vi "Enable-Disable SCISCAN Controls.vi"(7 "Enable-Disable SCISCAN Controls_Command":T2, 8 "Error In":errorcluster) -> (0 "Error Out":errorcluster)   [LabVIEW 2012]
doc: "SciScan 1.2 160622"
uses:
  Enable-Disable SCISCAN controls_Command.ctl
panel:
  out "Array":T1(array[cluster])
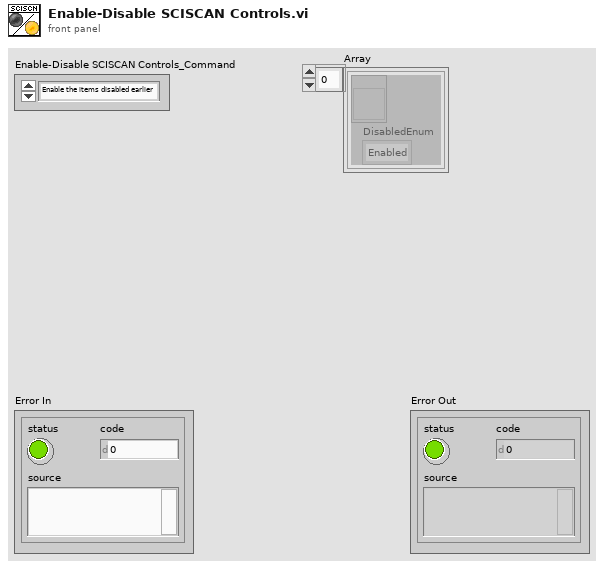
[diagram p1: front panel]
types:
  T1 = cluster{refnum<vi>, "DisabledEnum":enum8{"Enabled", "Disabled", "Disabled and Grayed Out"}}[]
  T2 = typedef "Enable-Disable SCISCAN controls_Command.ctl" = enum16{"Enable the items disabled earlier", "Disable", "Disable and Gray", "Enable all (except those in skip list)"}
  T3 = enum8{"Enabled", "Disabled", "Disabled and Grayed Out"}
  T4 = cluster{refnum<vi>, "DisabledEnum":enum8{"Enabled", "Disabled", "Disabled and Grayed Out"}}
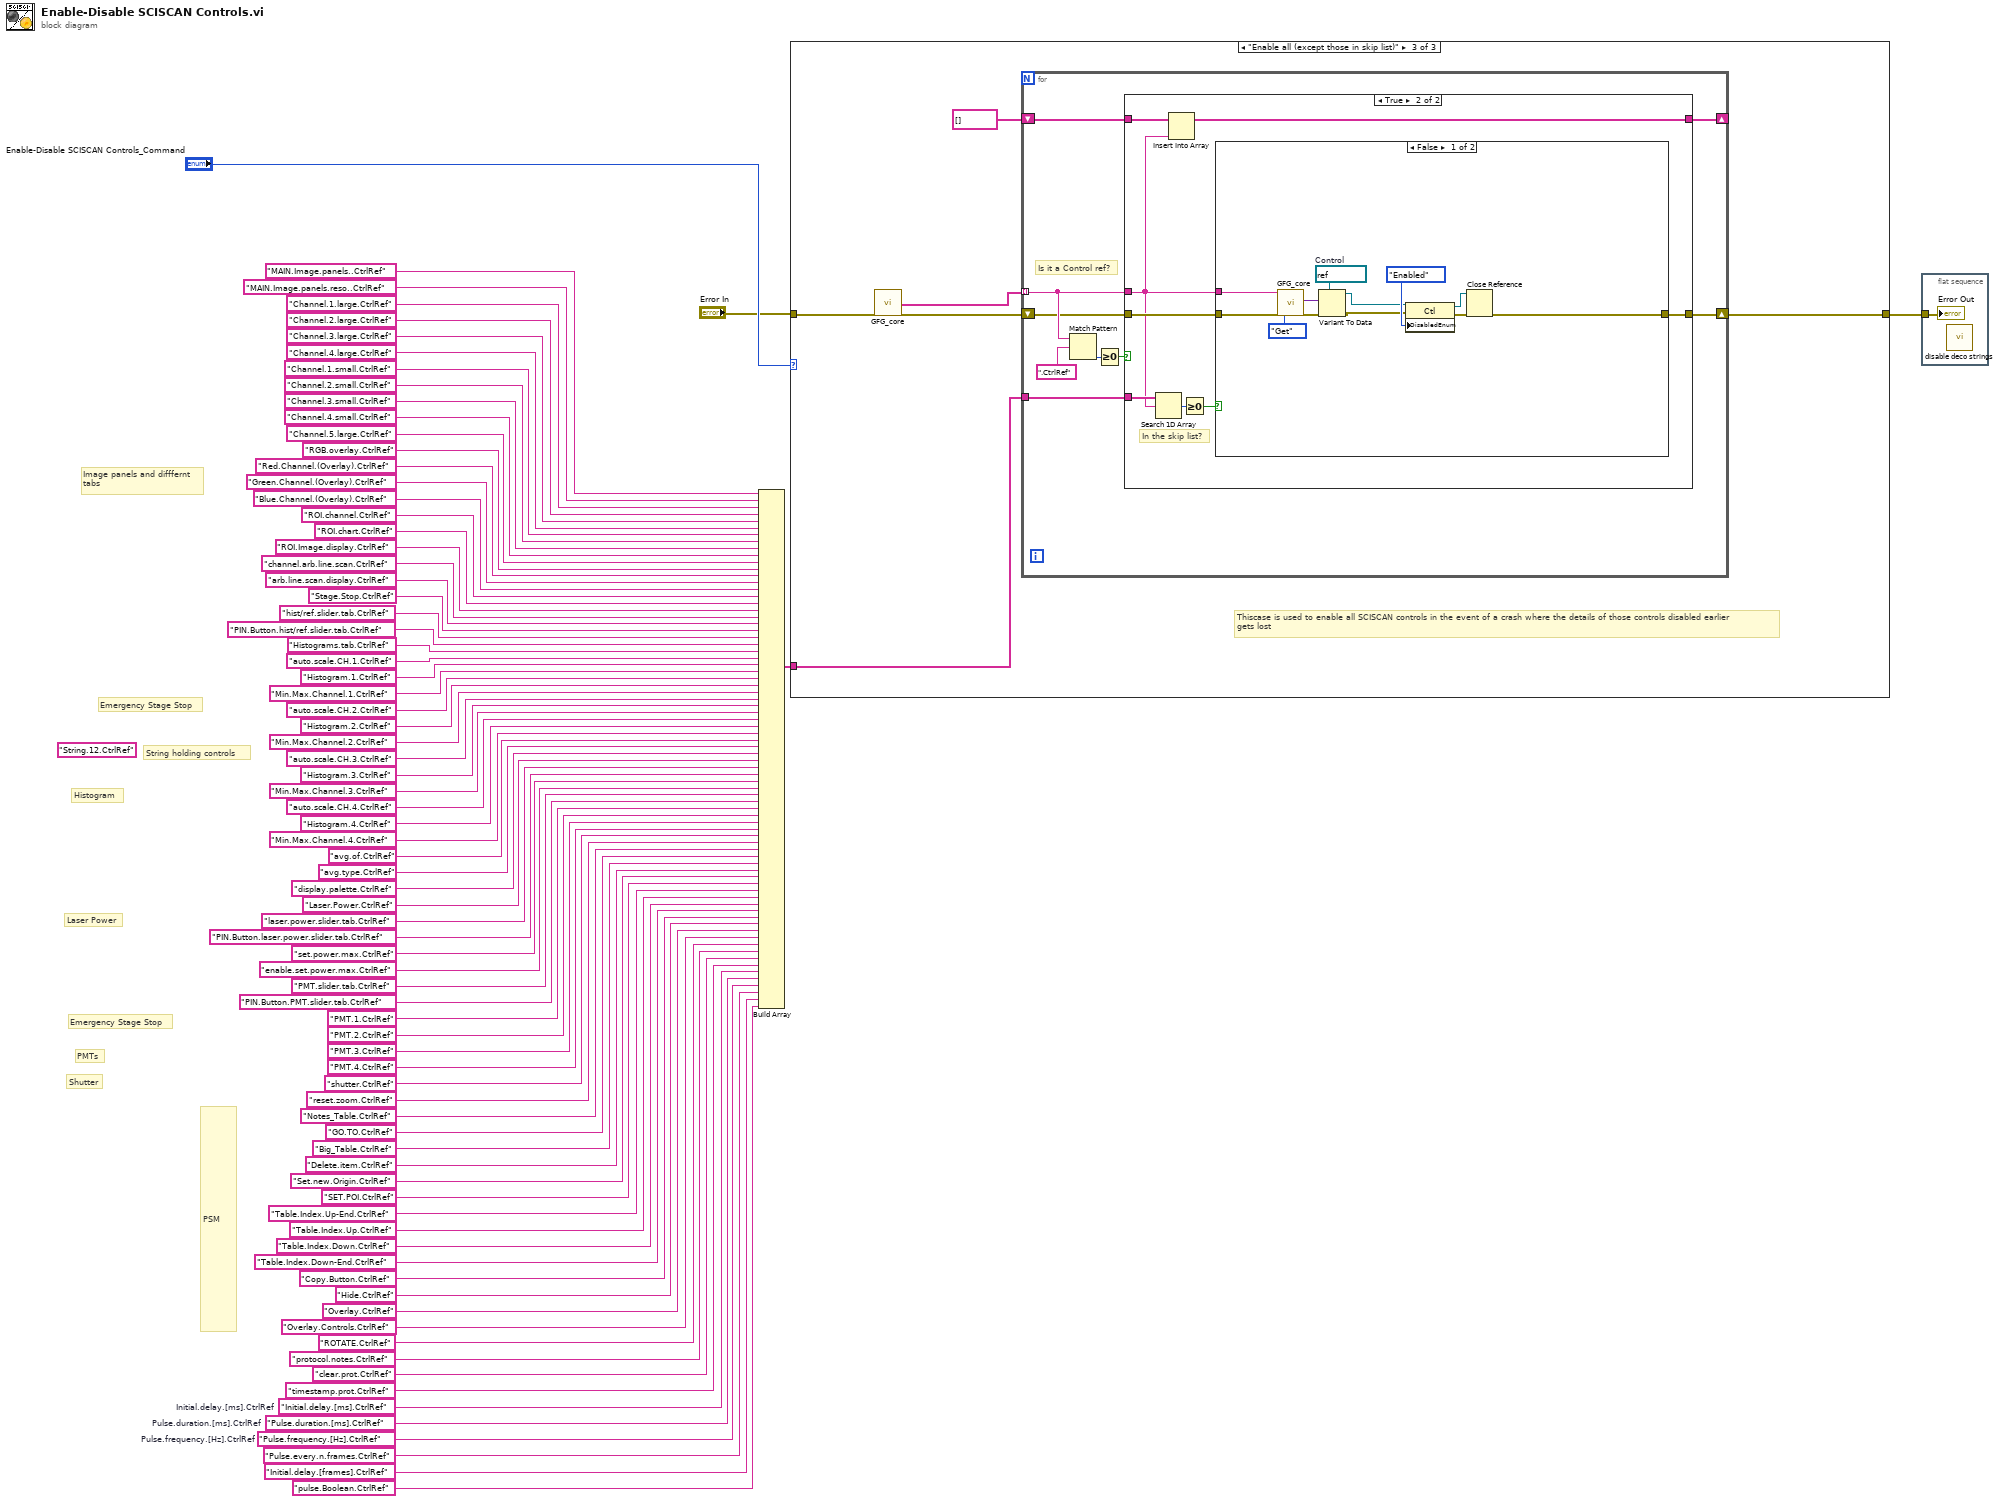
[diagram p0: block diagram]
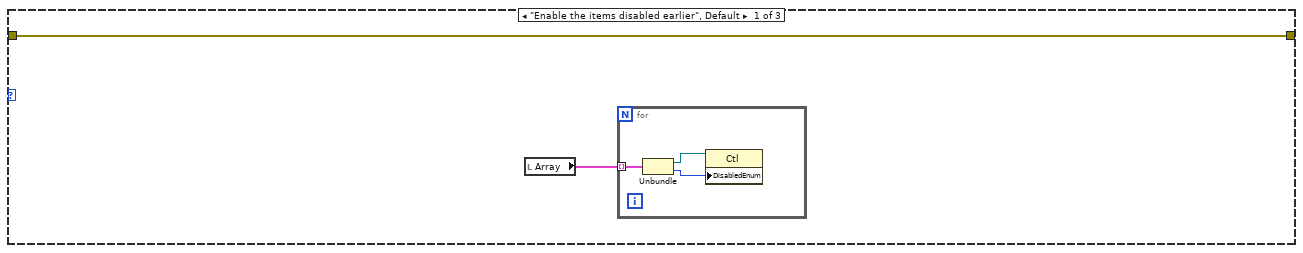
[diagram p2: hidden frame]
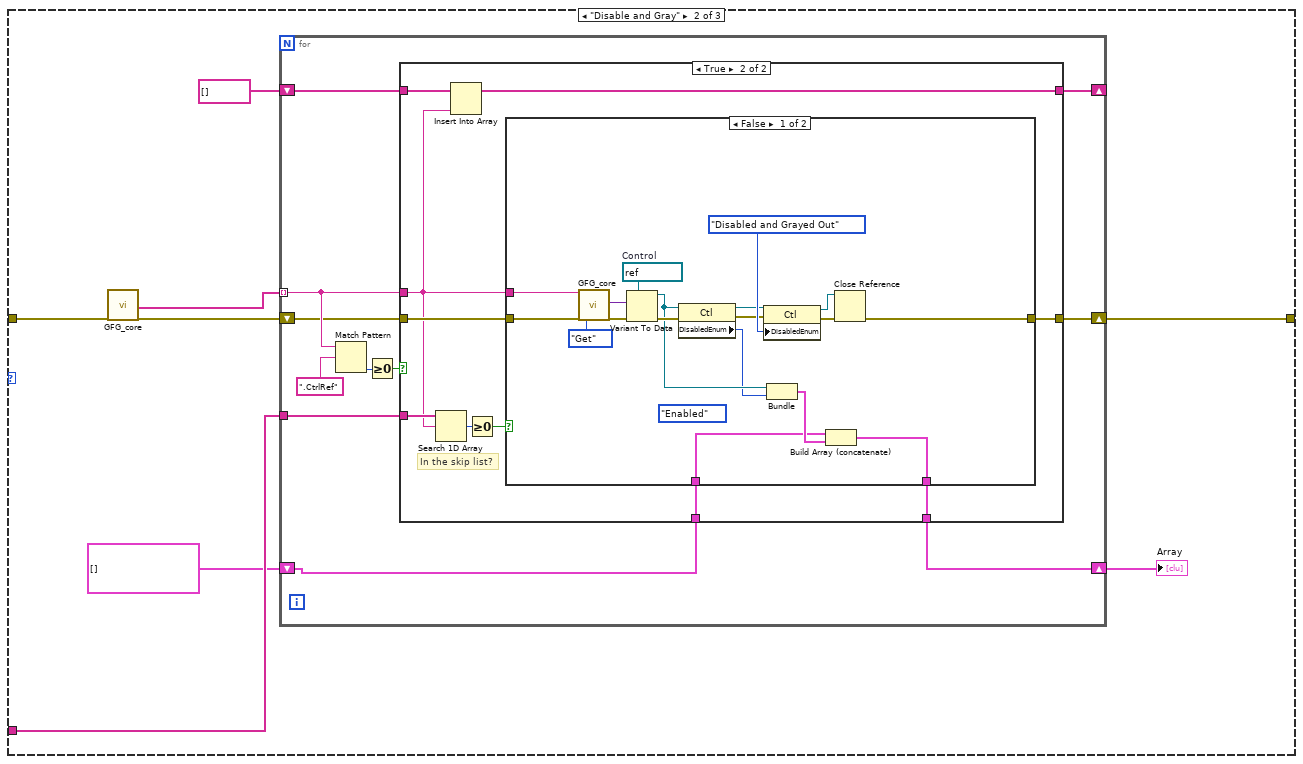
[diagram p3: hidden frame]
diagram:
  w4 = "Pulse.frequency.[Hz].CtrlRef"  # Pulse.frequency.[Hz].CtrlRef
  w5 = "Pulse.duration.[ms].CtrlRef"  # Pulse.duration.[ms].CtrlRef
  w6 = "Initial.delay.[ms].CtrlRef"  # Initial.delay.[ms].CtrlRef
  (unwired) "String.12.CtrlRef"
  # "PSM"
  # "Image panels and difffernt\ntabs"
  # "Histogram"
  # "Laser Power"
  # "PMTs"
  # "Shutter"
  # "Emergency Stage Stop"
  # "String holding controls"
  # "Emergency Stage Stop"
  n1 = Build Array("MAIN.Image.panels..CtrlRef", "MAIN.Image.panels.reso..CtrlRef", "Channel.1.large.CtrlRef", "Channel.2.large.CtrlRef", "Channel.3.large.CtrlRef", "Channel.4.large.CtrlRef", "Channel.1.small.CtrlRef", "Channel.2.small.CtrlRef", "Channel.3.small.CtrlRef", "Channel.4.small.CtrlRef", "Channel.5.large.CtrlRef", "RGB.overlay.CtrlRef", "Red.Channel.(Overlay).CtrlRef", "Green.Channel.(Overlay).CtrlRef", "Blue.Channel.(Overlay).CtrlRef", "ROI.channel.CtrlRef", "ROI.chart.CtrlRef", "ROI.Image.display.CtrlRef", "channel.arb.line.scan.CtrlRef", "arb.line.scan.display.CtrlRef", "Stage.Stop.CtrlRef", "hist/ref.slider.tab.CtrlRef", "PIN.Button.hist/ref.slider.tab.CtrlRef", "Histograms.tab.CtrlRef", "auto.scale.CH.1.CtrlRef", "Histogram.1.CtrlRef", "Min.Max.Channel.1.CtrlRef", "auto.scale.CH.2.CtrlRef", "Histogram.2.CtrlRef", "Min.Max.Channel.2.CtrlRef", "auto.scale.CH.3.CtrlRef", "Histogram.3.CtrlRef", "Min.Max.Channel.3.CtrlRef", "auto.scale.CH.4.CtrlRef", "Histogram.4.CtrlRef", "Min.Max.Channel.4.CtrlRef", "avg.of.CtrlRef", "avg.type.CtrlRef", "display.palette.CtrlRef", "Laser.Power.CtrlRef", "laser.power.slider.tab.CtrlRef", "PIN.Button.laser.power.slider.tab.CtrlRef", "set.power.max.CtrlRef", "enable.set.power.max.CtrlRef", "PMT.slider.tab.CtrlRef", "PIN.Button.PMT.slider.tab.CtrlRef", "PMT.1.CtrlRef", "PMT.2.CtrlRef", "PMT.3.CtrlRef", "PMT.4.CtrlRef", "shutter.CtrlRef", "reset.zoom.CtrlRef", "Notes_Table.CtrlRef", "GO.TO.CtrlRef", "Big_Table.CtrlRef", "Delete.item.CtrlRef", "Set.new.Origin.CtrlRef", "SET.POI.CtrlRef", "Table.Index.Up-End.CtrlRef", "Table.Index.Up.CtrlRef", "Table.Index.Down.CtrlRef", "Table.Index.Down-End.CtrlRef", "Copy.Button.CtrlRef", "Hide.CtrlRef", "Overlay.CtrlRef", "Overlay.Controls.CtrlRef", "ROTATE.CtrlRef", "protocol.notes.CtrlRef" ("element"), "clear.prot.CtrlRef" ("element"), "timestamp.prot.CtrlRef" ("element"), w6, w5, w4, "Pulse.every.n.frames.CtrlRef", "Initial.delay.[frames].CtrlRef", "pulse.Boolean.CtrlRef" ("Variable Name in")) -> (w79:string[])
  n2 = case shown="\"Enable all (except those in skip list)\"" "Enable-Disable SCISCAN Controls_Command" {
    tunnel: w79 -> [_ w92 w142]
    tunnel: [w81 w86 w139] -> w26
    tunnel: "Error In" -> [w81 w87 w138]
    frame "Enable the items disabled earlier", Default {
      n3 = local read "Array"() -> (w82:T1)
      n4 = for {
        tunnel: w82 -> [w85] mode=indexing
        n5 = Unbundle(w85) -> (w84:refnum<vi>, "DisabledEnum"=w83:T3)
        n6 = property class="Ctl"(reference=w84, "DisabledEnum"=w83) -> ()  [unwired: 1 in, 2 out]
      }
    }
    frame "Disable and Gray" {
      n7 = call "GFG_core.vi"("error in (no error)"=w87) -> ("All Variable Names Out"=w93:string[], "error out"=w91:errorcluster)  [unwired: 12 in, 5 out]
      n8 = for {
        tunnel: w93 -> [w103] mode=indexing
        tunnel: w92 -> [w102]
        shift-right: [w98] -> w86
        shift-left: w91 -> [w99]
        shift-right: [w96] -> _
        shift-left: string[] [] -> [w97]
        shift-right: [w94] -> w89
        shift-left: T1 [] -> [w95]
        n9 = Match Pattern(string=w103, regular expression=".CtrlRef" ("string")) -> (offset past match=w101:i32)  [unwired: 1 in, 3 out]
        n10 = Greater Or Equal To 0?(x=w101) -> (x >= 0?=w100:bool)
        n11 = case shown="True" w100 {
          tunnel: w103 -> [_ w111]
          tunnel: w102 -> [_ w117]
          tunnel: w99 -> [w107 w114]
          tunnel: [w107 w113] -> w98
          tunnel: w97 -> [w106 w112]
          tunnel: [w106 w110] -> w96
          tunnel: w95 -> [w105 w109]
          tunnel: [w105 w108] -> w94
          frame False {
          }
          frame True {
            # "In the skip list?"
            n12 = Search 1D Array(1D array=w117, element=w111) -> (index of element=w116:i32)  [unwired: 1 in]
            n13 = Insert Into Array(array=w112, new element=w111) -> (w110:string[])  [unwired: 1 in]
            n14 = Greater Or Equal To 0?(x=w116) -> (x >= 0?=w115:bool)
            n15 = case shown="False" w115 {
              tunnel: w111 -> [w135 _]
              tunnel: w114 -> [w134 w137]
              tunnel: [w133 w137] -> w113
              tunnel: w109 -> [w119 w136]
              tunnel: [w121 w136] -> w108
              frame False {
                (unwired) T3."Enabled" ("Disabled")
                w131 = refnum<vi> refnum  # Control
                n16 = call "GFG_core.vi"("Variable Name in"=w135, "error in (no error)"=w134, "Action"=enum16{"Init", "Set", "Get", "Clear"}."Get") -> ("Variant Out"=w130:variant, "error out"=w128:errorcluster)  [unwired: 10 in, 5 out]
                n17 = Variant To Data(error in=w128, type=w131, Variant=w130) -> (data=w122:refnum<vi>, error out=w125:errorcluster)
                n18 = property class="Ctl"(reference=w122, error in=w125) -> (reference out=w124:refnum<vi>, error out=w123:errorcluster, "DisabledEnum"=w118:T3)
                n19 = property class="Ctl"(reference=w124, error in=w123, "DisabledEnum"=T3."Disabled and Grayed Out" ("Disabled")) -> (reference out=w126:refnum<vi>, error out=w127:errorcluster)
                n20 = Bundle(w122, "DisabledEnum"=w118) -> (w120:T4)  [unwired: 1 in]
                n21 = Build Array (concatenate)(w119, w120) -> (w121:T1)
                n22 = Close Reference(reference=w126, error in (no error)=w127) -> (error out=w133:errorcluster)
              }
              frame True {
              }
            }
          }
        }
      }
      "Array" <- w89
    }
    frame "Enable all (except those in skip list)" {
      # "Thiscase is used to enable all SCISCAN controls in the event of a crash where the details of those controls disabled earlier\ngets lost"
      n23 = call "GFG_core.vi"("error in (no error)"=w138) -> ("All Variable Names Out"=w143:string[], "error out"=w141:errorcluster)  [unwired: 12 in, 5 out]
      n24 = for {
        tunnel: w143 -> [w151] mode=indexing
        tunnel: w142 -> [w150]
        shift-right: [w146] -> w139
        shift-left: w141 -> [w147]
        shift-right: [w144] -> _
        shift-left: string[] [] -> [w145]
        # "Is it a Control ref?"
        n25 = Match Pattern(string=w151, regular expression=".CtrlRef" ("string")) -> (offset past match=w149:i32)  [unwired: 1 in, 3 out]
        n26 = Greater Or Equal To 0?(x=w149) -> (x >= 0?=w148:bool)
        n27 = case shown="True" w148 {
          tunnel: w151 -> [_ w156]
          tunnel: w150 -> [_ w162]
          tunnel: w147 -> [w154 w159]
          tunnel: [w154 w158] -> w146
          tunnel: w145 -> [w153 w157]
          tunnel: [w153 w155] -> w144
          frame False {
          }
          frame True {
            # "In the skip list?"
            n28 = Search 1D Array(1D array=w162, element=w156) -> (index of element=w161:i32)  [unwired: 1 in]
            n29 = Insert Into Array(array=w157, new element=w156) -> (w155:string[])  [unwired: 1 in]
            n30 = Greater Or Equal To 0?(x=w161) -> (x >= 0?=w160:bool)
            n31 = case shown="False" w160 {
              tunnel: w156 -> [w174 _]
              tunnel: w159 -> [w173 w175]
              tunnel: [w172 w175] -> w158
              frame False {
                w170 = refnum<vi> refnum  # Control
                n32 = call "GFG_core.vi"("Variable Name in"=w174, "error in (no error)"=w173, "Action"=enum16{"Init", "Set", "Get", "Clear"}."Get") -> ("Variant Out"=w169:variant, "error out"=w167:errorcluster)  [unwired: 10 in, 5 out]
                n33 = Variant To Data(error in=w167, type=w170, Variant=w169) -> (data=w164:refnum<vi>, error out=w163:errorcluster)
                n34 = property class="Ctl"(reference=w164, error in=w163, "DisabledEnum"=T3."Enabled" ("Disabled")) -> (reference out=w165:refnum<vi>, error out=w166:errorcluster)
                n35 = Close Reference(reference=w165, error in (no error)=w166) -> (error out=w172:errorcluster)
              }
              frame True {
              }
            }
          }
        }
      }
    }
  }
  n36 = flat-sequence {
    tunnel: w26 -> [w176]
    frame #0 {
      n37 = call "disable deco strings.vi"() -> ()  [unwired: 11 in, 1 out]
      "Error Out" <- w176
    }
  }
